vi "Write PID Settings.vi"(0 "VISA Session In":refnum<visa-resource-name>="Alicat", 2 "PID Loop Settings":T1={"PID Type"=enum."PDF", "Valve Offset"=18000}, 3 "error in":errorcluster, 4 "Unit ID (A)":string="A") -> (7 "VISA Session Out":refnum<visa-resource-name>, 10 "error out":errorcluster)   [LabVIEW 2019]
doc: "Writes the PID loop type and the valve offset options to the connected Alicat device. PID loop type is default PDF for single valve units and can only be PD2I if using a dual valve unit. The valve offset effects the initial kick to the valve to begin flowing from a hard zero (contact Alicat for default values if not functioning properly: (520) 290-6060 or info@alicat.com)."
panel:
  # "Alterations to either of these should be performed with care, as they can drastically alter how the controller performs"
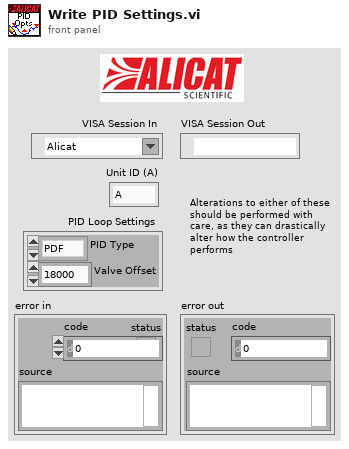
[diagram p1: front panel]
types:
  T1 = cluster{"PID Type":enum8{"PDF", "PD2I"}, "Valve Offset":i32}
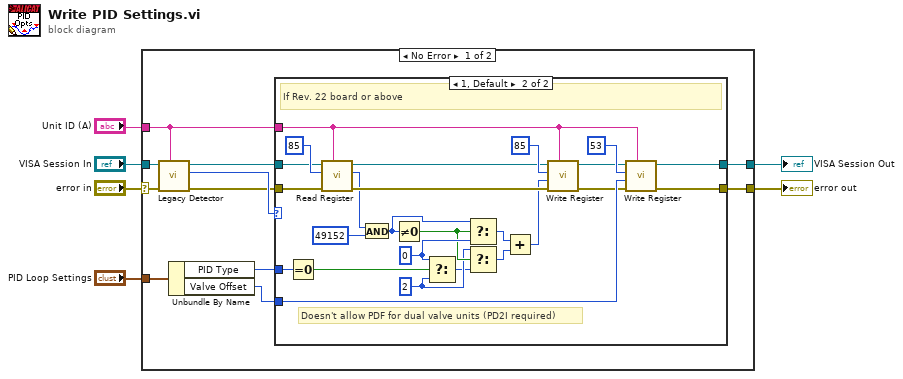
[diagram p0: block diagram]
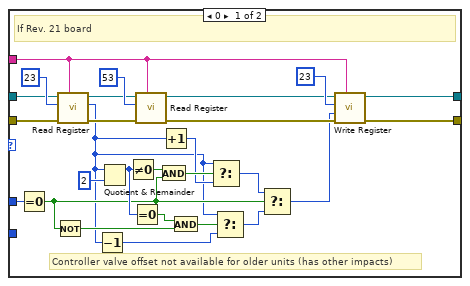
[diagram p2: hidden frame]
diagram:
  n1 = case shown="No Error" "error in" {
    selector: "error in" -> [w16 w70]
    tunnel: [w15 w70] -> w6
    tunnel: [w14 w71] -> w5
    tunnel: "VISA Session In" -> [w17 w71]
    tunnel: "Unit ID (A)" -> [w7 _]
    tunnel: "PID Loop Settings" -> [w13 _]
    frame No Error {
      n2 = call "Legacy Detector.vi"("Unit ID (A)"=w7, "error in"=w16, "VISA Session In"=w17) -> ("error out"=w10:errorcluster, "Legacy Status"=w12:u8, "VISA Session Out"=w11:refnum<visa-resource-name>)  [unwired: 6 in]
      n3 = Unbundle By Name(w13) -> ("PID Type"=w9:enum8{"PDF", "PD2I"}, "Valve Offset"=w8:i32)
      n4 = case shown="1, Default" w12 {
        tunnel: [w41 w50] -> w15
        tunnel: [w42 w49] -> w14
        tunnel: w11 -> [w39 w66]
        tunnel: w10 -> [w38 w65]
        tunnel: w9 -> [w32 w60]
        tunnel: w8 -> [_ w55]
        tunnel: w7 -> [w18 w46]
        frame 0 {
          # "Controller valve offset not available for older units (has other impacts)"
          # "If Rev. 21 board"
          n5 = Equal To 0?(x=w32) -> (x = 0?=w22:bool)
          n6 = Not(x=w22) -> (.not. x?=w21:bool)
          n7 = call "Read Register.vi"("Unit ID (A)"=w18, "error in"=w38, "Register address"=u16 23, "VISA Session In"=w39) -> ("error out"=w35:errorcluster, "Register Value (I32)"=w20:i32, "VISA Session Out"=w36:refnum<visa-resource-name>)  [unwired: 5 in]
          n8 = Decrement(x=w20) -> (x-1=w27:i32)
          n9 = Quotient & Remainder(x=w20, y=2) -> (x-y*floor(x/y)=w23:i32)  [unwired: 1 out]
          n10 = Not Equal To 0?(x=w23) -> (x != 0?=w31:bool)
          n11 = Equal To 0?(x=w23) -> (x = 0?=w24:bool)
          n12 = call "Read Register.vi"("Unit ID (A)"=w18, "error in"=w35, "Register address"=u16 53, "VISA Session In"=w36) -> ("error out"=w34:errorcluster, "VISA Session Out"=w33:refnum<visa-resource-name>)  [unwired: 5 in, 1 out]
          n13 = And(x=w31, y=w22) -> (x .and. y?=w30:bool)
          n14 = Increment(x=w20) -> (x+1=w29:i32)
          n15 = And(x=w24, y=w21) -> (x .and. y?=w26:bool)
          n16 = Select(t=w20, s=w30, f=w29) -> (s? t:f=w28:i32)
          n17 = Select(t=w20, s=w26, f=w27) -> (s? t:f=w25:i32)
          n18 = Select(t=w28, s=w22, f=w25) -> (s? t:f=w19:i32)
          n19 = call "Write Register.vi"("Unit ID (A)"=w18, "error in"=w34, "Register Value"=w19, "Register address"=u16 23, "VISA Session In"=w33) -> ("error out"=w41:errorcluster, "VISA Session Out"=w42:refnum<visa-resource-name>)  [unwired: 4 in, 1 out]
        }
        frame 1, Default {
          w53 = 2 ("f")
          w58 = 0 ("f")
          # "Doesn't allow PDF for dual valve units (PD2I required)"
          # "If Rev. 22 board or above"
          n20 = Equal To 0?(x=w60) -> (x = 0?=w59:bool)
          n21 = call "Read Register.vi"("Unit ID (A)"=w46, "error in"=w65, "Register address"=u16 85, "VISA Session In"=w66) -> ("error out"=w64:errorcluster, "Register Value (I32)"=w62:i32, "VISA Session Out"=w63:refnum<visa-resource-name>)  [unwired: 5 in]
          n22 = And(x=w62, y=49152) -> (x .and. y?=w45:i32)
          n23 = Not Equal To 0?(x=w45) -> (x != 0?=w54:bool)
          n24 = Select(t=w58, s=w59, f=w53) -> (s? t:f=w52:i32)
          n25 = Select(t=w45, s=w54, f=w58) -> (s? t:f=w57:i32)
          n26 = Select(t=w53, s=w54, f=w52) -> (s? t:f=w51:i32)
          n27 = Add(x=w57, y=w51) -> (x+y=w56:i32)
          n28 = call "Write Register.vi"("Unit ID (A)"=w46, "error in"=w64, "Register Value"=w56, "Register address"=u16 85, "VISA Session In"=w63) -> ("error out"=w47:errorcluster, "VISA Session Out"=w48:refnum<visa-resource-name>)  [unwired: 4 in, 1 out]
          n29 = call "Write Register.vi"("Unit ID (A)"=w46, "error in"=w47, "Register Value"=w55, "Register address"=u16 53, "VISA Session In"=w48) -> ("error out"=w50:errorcluster, "VISA Session Out"=w49:refnum<visa-resource-name>)  [unwired: 4 in, 1 out]
        }
      }
    }
    frame Error {
    }
  }
  "error out" <- w6
  "VISA Session Out" <- w5
